vi "Read Broadcast Action.vi"(8 "error in (no error)":errorcluster, 11 "EventsAbstract in":refnum<class "EventsAbstract.lvclass">) -> (0 "error out":errorcluster, 2 "Broadcast Action":bool, 3 "EventsAbstract out":refnum<class "EventsAbstract.lvclass">)   [LabVIEW 2019, in "EventsAbstract.lvclass"]
uses:
  EventsAbstract.lvclass
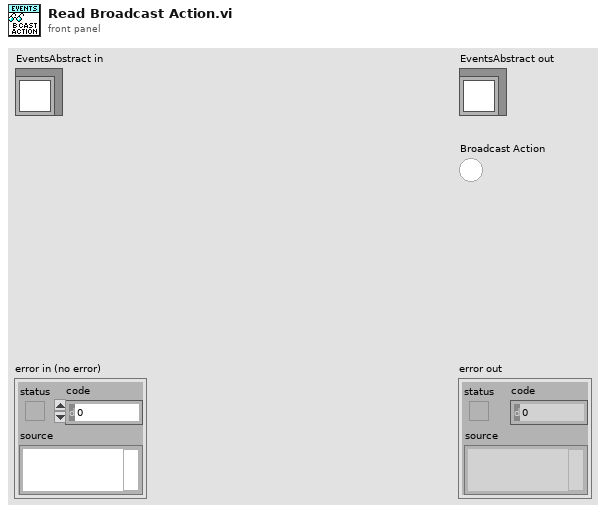
[diagram p1: front panel]
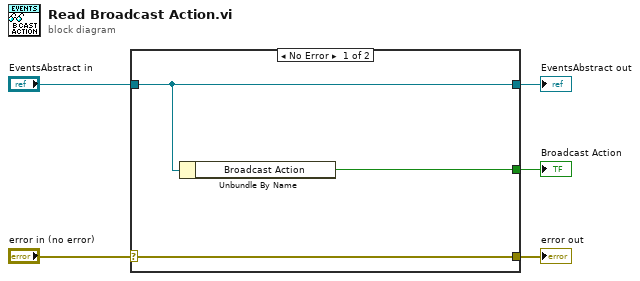
[diagram p0: block diagram]
diagram:
  n1 = case shown="No Error" "error in (no error)" {
    selector: "error in (no error)" -> [w8 w9]
    tunnel: [w8 w9] -> w4
    tunnel: [w7 w10] -> w2
    tunnel: "EventsAbstract in" -> [w7 w10]
    tunnel: [w6 _] -> w1
    frame No Error {
      n2 = Unbundle By Name(w7) -> ("Broadcast Action"=w6:bool)
    }
    frame Error {
    }
  }
  "error out" <- w4
  "EventsAbstract out" <- w2
  "Broadcast Action" <- w1
